vi "Global_Cube_Steering.vi"() -> ()   [LabVIEW 2017]
panel:
  in  "Max speed":dbl
  in  "Deadband":dbl
  in  "Scale Factor":dbl
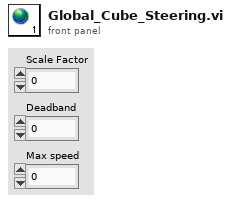
[diagram p1: front panel]
diagram:
